vi "FacadeResizable1DArray(U16).vi"(0 "Data In":T4, 2 "Display State In":T2, 3 "Container State":T3) -> (6 "Data Out":T4, 7 "Display State Out":T2, 8 "Action":T1)   [LabVIEW 2011, in "Resizable1DArray(U16).xctl"]
uses:
  <vilib>/_probes/SAPHIR/ViBox - Probes/Resizable1DArray/Resizable1DArray(U16)/Resizable1DArray(U16).xctl
  <vilib>/_probes/SAPHIR/ViBox - Probes/Resizable1DArray/Resizable1DArray(U16)/DataResizable1DArray(U16).ctl
  <vilib>/_xctls/Container State.ctl
  <vilib>/_probes/SAPHIR/ViBox - Probes/Resizable1DArray/Resizable1DArray(U16)/StateResizable1DArray(U16).ctl
  <vilib>/_xctls/Action.ctl
  <vilib>/_xctls/XControlSupport.lvlib
panel:
  in  "Format":string caption="Format :"
  out "Numeric":u16
  out "[U16]":u16[](array[numeric])
  # "Display Options"
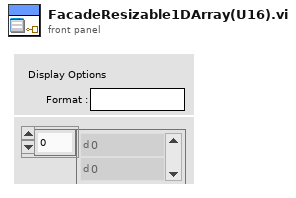
[diagram p1: front panel]
types:
  T1 = typedef "XControlSupport.lvlib/Action.ctl" = cluster{"Data Changed?":bool, "State Changed?":bool, "Action Name":string}
  T2 = typedef "Resizable1DArray(U16).xctl/StateResizable1DArray(U16).ctl" = cluster{"Height":u32}
  T3 = typedef "XControlSupport.lvlib/Container State.ctl" = cluster{"Indicator?":bool, "Run Mode?":bool, " Refnum":refnum<vi>}
  T4 = typedef "Resizable1DArray(U16).xctl/DataResizable1DArray(U16).ctl" = u16[]
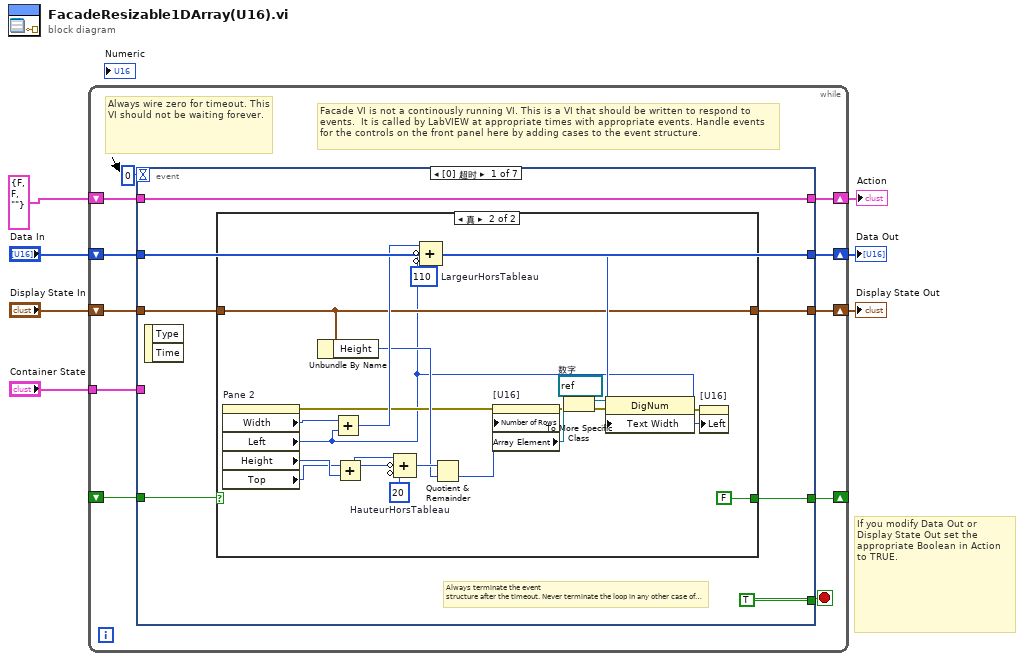
[diagram p0: block diagram]
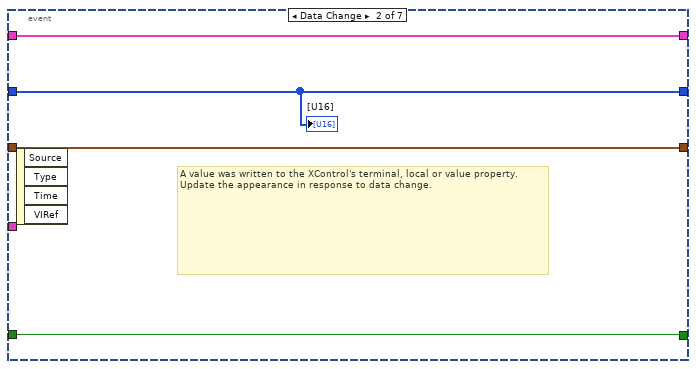
[diagram p3: hidden frame]
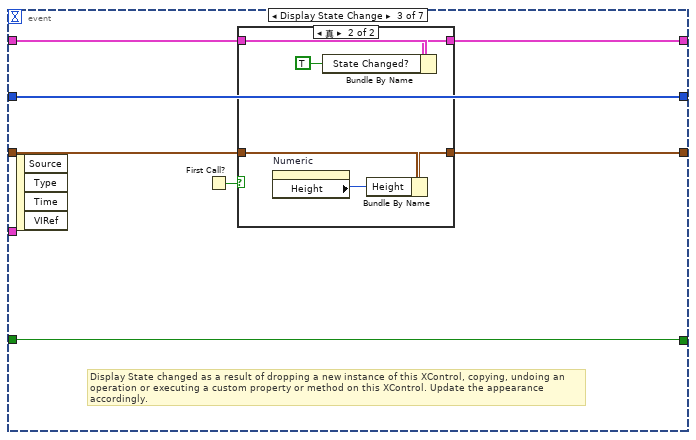
[diagram p4: hidden frame]
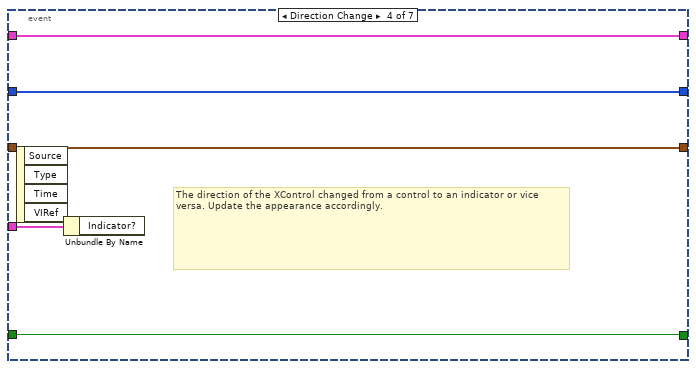
[diagram p6: hidden frame]
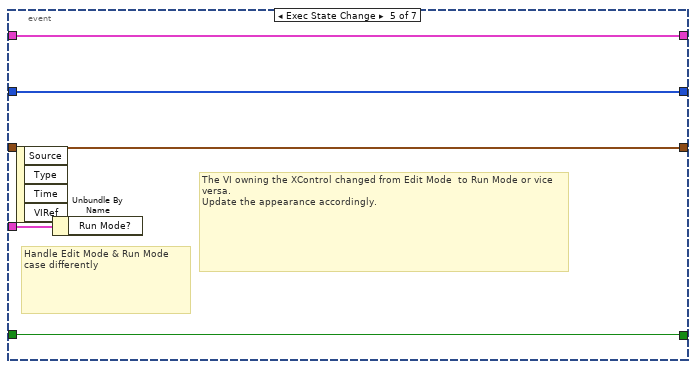
[diagram p7: hidden frame]
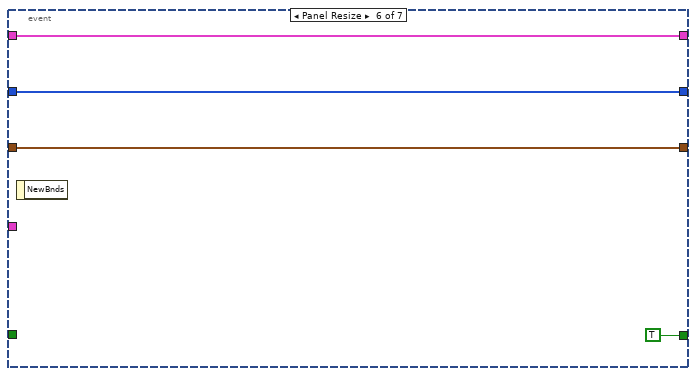
[diagram p8: hidden frame]
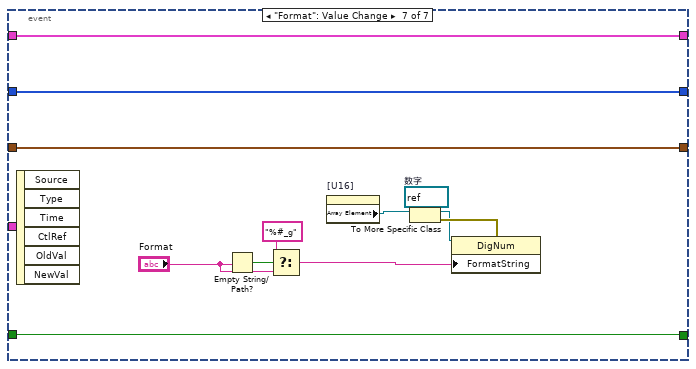
[diagram p9: hidden frame]
diagram:
  # "If you modify Data Out or\nDisplay State Out set the\nappropriate Boolean in Action\nto TRUE."
  n1 = while {
    shift-right: [w17] -> w5
    shift-left: "Display State In" -> [w18]
    tunnel: "Container State" -> [w14]
    shift-right: [w12] -> w7
    shift-left: "Data In" -> [w13]
    shift-right: [w10] -> w3
    shift-left: T1 {"Data Changed?"=FALSE, "State Changed?"=FALSE, "Action Name"=""} ("Action") -> [w11]
    shift-right: [w8] -> _
    shift-left: _ -> [w9]
    stop <- w16 stop-if-true
    # "Facade VI is not a continously running VI. This is a VI that should be written to respond to events.  It is called by LabVIEW at appropriate times with appropriate events. Handle events for the controls on the front panel here by adding cases to the event structure."
    # "Always wire zero for timeout. This\nVI should not be waiting forever."
    n2 = event shown="[0] 超时" {
      selector: _ -> [_ _ _ _ _ _ _]
      dyn-events: _ -> [_ _ _ _ _ _ _]
      timeout: 0 -> [_ _ _ _ _ _ _]
      tunnel: w18 -> [w22 w52 w56 w71 w76 w80 w90]
      tunnel: [w21 w52 w55 w71 w76 w80 w90] -> w17
      tunnel: [TRUE _ _ _ _ _ _] -> w16
      tunnel: w14 -> [_ _ _ w72 w77 _ _]
      tunnel: w13 -> [w23 w50 w59 w70 w75 w81 w91]
      tunnel: [w23 w50 w59 w70 w75 w81 w91] -> w12
      tunnel: [w24 w51 w53 w69 w74 w79 w92] -> w10
      tunnel: w11 -> [w24 w51 w54 w69 w74 w79 w92]
      tunnel: w9 -> [w20 w49 w58 w68 w73 _ w93]
      tunnel: [w19 w49 w58 w68 w73 TRUE w93] -> w8
      event Timeout {
        # "Always terminate the event\nstructure after the timeout. Never terminate the loop in any other case of the event structure."
        n3 = event-data() -> ()  [unwired: 3 out]
        n4 = case shown="真" w20 {
          selector: w20 -> [w26 _]
          tunnel: w22 -> [w27 w36]
          tunnel: [w27 w36] -> w21
          tunnel: [w26 FALSE] -> w19
          frame False {
          }
          frame True {
            w44 = refnum<vi> refnum  # 数字
            w46 = i16 20  # HauteurHorsTableau
            w45 = i16 110  # LargeurHorsTableau
            n5 = property on="Pane 2" class="Pane"() -> (error out=w32:errorcluster, "Width"=w31:u32, "Left"=w30:i32, "Height"=w29:u32, "Top"=w28:i32)  [unwired: 2 in, 1 out]
            n6 = Unbundle By Name(w36) -> ("Height"=w34:u32)
            n7 = Add(x=w31, y=w30) -> (x+y=w47:u32)
            n8 = Add(x=w28, y=w29) -> (x+y=w37:u32)
            n9 = Compound Arithmetic op=ADD(w37, invert w28, invert w46) -> (w41:u32)
            n10 = Compound Arithmetic op=ADD(w47, invert w30, invert w45) -> (w48:u32)
            n11 = Quotient & Remainder(x=w41, y=w34) -> (floor(x/y)=w35:u32)  [unwired: 1 out]
            n12 = property on="[U16]" class="Arr (严格)"(error in=w32, "Number of Rows"=w35) -> (error out=w40:errorcluster, "Array Element"=w42:refnum<vi>)  [unwired: 1 in, 1 out]
            n13 = To More Specific Class(target class=w44, reference=w42, error in=w40) -> (specific class reference=w43:refnum<vi>, error out=w39:errorcluster)
            n14 = property class="DigNum"(reference=w43, error in=w39, "Text Width"=w48) -> (error out=w38:errorcluster)  [unwired: 1 out]
            n15 = property on="[U16]" class="Arr (严格)"(error in=w38, "Left"=w30) -> ()  [unwired: 1 in, 2 out]
          }
        }
      }
      event Data Change {
        # "A value was written to the XControl's terminal, local or value property.\nUpdate the appearance in response to data change."
        n16 = event-data() -> ()  [unwired: 5 out]
        "[U16]" <- w50
      }
      event Display State Change {
        # "Display State changed as a result of dropping a new instance of this XControl, copying, undoing an operation or executing a custom property or method on this XControl. Update the appearance accordingly."
        n17 = event-data() -> ()  [unwired: 5 out]
        n18 = First Call?() -> (First Call?: T/F=w57:bool)
        n19 = case shown="真" w57 {
          tunnel: w56 -> [w61 w67]
          tunnel: [w61 w66] -> w55
          tunnel: w54 -> [w60 w64]
          tunnel: [w60 w63] -> w53
          frame False {
          }
          frame True {
            n20 = property on="Numeric" class="DigNum (严格)"() -> ("Height"=w65:u32)  [unwired: 2 in, 2 out]
            n21 = Bundle By Name(cluster=w64, "State Changed?"=TRUE) -> (w63:T1)
            n22 = Bundle By Name(cluster=w67, "Height"=w65) -> (w66:T2)
          }
        }
      }
      event Direction Change {
        # "The direction of the XControl changed from a control to an indicator or vice versa. Update the appearance accordingly."
        n23 = event-data() -> ()  [unwired: 5 out]
        n24 = Unbundle By Name(w72) -> ()  [unwired: 1 out]
      }
      event Exec State Change {
        # "The VI owning the XControl changed from Edit Mode  to Run Mode or vice versa.\nUpdate the appearance accordingly."
        # "Handle Edit Mode & Run Mode\ncase differently"
        n25 = event-data() -> ()  [unwired: 5 out]
        n26 = Unbundle By Name(w77) -> ()  [unwired: 1 out]
      }
      event Panel Resize {
        n27 = event-data() -> ()  [unwired: 2 out]
      }
      event "Format": Value Change {
        w83 = refnum<vi> refnum  # 数字
        n28 = event-data() -> ()  [unwired: 7 out]
        n29 = Empty String/Path?(string/path="Format") -> (empty?=w87:bool)
        n30 = Select(t="%#_g", s=w87, f="Format") -> (s? t:f=w89:string)
        n31 = property on="[U16]" class="Arr (严格)"() -> ("Array Element"=w86:refnum<vi>)  [unwired: 2 in, 2 out]
        n32 = To More Specific Class(target class=w83, reference=w86) -> (specific class reference=w84:refnum<vi>, error out=w85:errorcluster)  [unwired: 1 in]
        n33 = property class="DigNum"(reference=w84, error in=w85, "FormatString"=w89) -> ()  [unwired: 2 out]
      }
    }
  }
  "Display State Out" <- w5
  "Data Out" <- w7
  "Action" <- w3
